vi "PTFE Test.vi"() -> ()   [LabVIEW 2015]
uses:
  Controls/Vacuum State Enumerator.ctl
  <vilib>/Platform/TimedLoop/XDataNode/timing_clust.ctl
  <vilib>/Platform/TimedLoop/XDataNode/nitl_modes.ctl
  <vilib>/Platform/TimedLoop/XDataNode/wakeup.ctl
  <vilib>/platform/TimedLoop/XDataNode/XDataNode.xnode
  <vilib>/Platform/TimedLoop/XDataNode/XDNodeRunTimeDep.lvlib
panel:
  out "x/y":dbl(slide) scale=0.0..1.0
  in  "Enable":bool
  in  "Waveform Graph 3":dbl[](graph)=array[50278 elements]
  out "Waveform Graph 2":dbl[](graph)
  in  "Vacuum State":T1=enum."Unknown"
  out "Valve":bool
  in  "Numeric":dbl
  out "Waveform Graph":dbl[](graph)
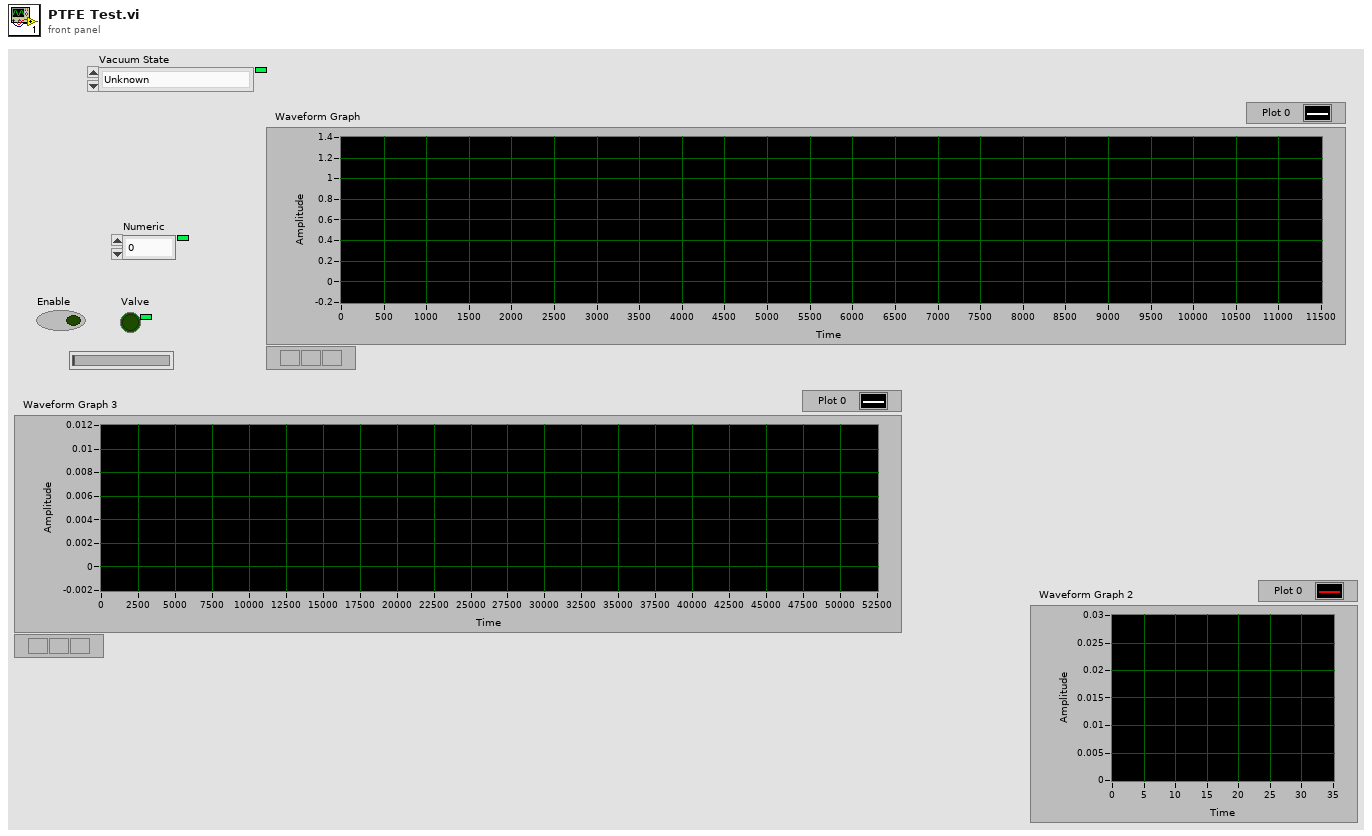
[diagram p1: front panel]
types:
  T1 = typedef "Vacuum State Enumerator.ctl" = enum16{"Pressure Rising", "Plateau", "Pressure Dropping", "Valley", "Low Valley", "Leak", "Unknown"}
  T2 = typedef "XDNodeRunTimeDep.lvlib/timing_clust.ctl" = cluster{"Expected End [f-1]":u64, "Actual End [f-1]":u64, "Finished Late? [f-1]":bool, "Expected End [i-1]":u64, "Actual End [i-1]":u64, "Finished Late? [i-1]":bool, "Expected Start [i]":u64, "Actual Start [i]":u64, "Expected Start [f]":u64, "Actual Start [f]":u64, "Source Name":string, "Structure Name":string, "Period":i64, "Deadline":i64, "Offset":i64, "Start":i64, "Priority":i32, "Timeout":i32, "Mode":T3, "Wakeup Reason":T4, "Error":errorcluster, "Source Type":string, "Secondary Source Type":string, "Global End Time":u64, "Global Start Time":u64, "Frame Duration":u64, "Iteration Duration":u64, "Assigned CPU":i32, "I/O Scan Engine Mode":u32}
  T3 = typedef "XDNodeRunTimeDep.lvlib/nitl_modes.ctl" = enum32{"No Change", "Process missed periods, maintain original phase", "Discard missed periods, maintain original phase", "Process missed periods, ignore original phase", "Discard missed periods, ignore original phase"}
  T4 = typedef "XDNodeRunTimeDep.lvlib/wakeup.ctl" = enum32{"Normal", "Aborted", "Asynchronous wakeup", "Timing source error", "Timed loop error", "Timeout"}
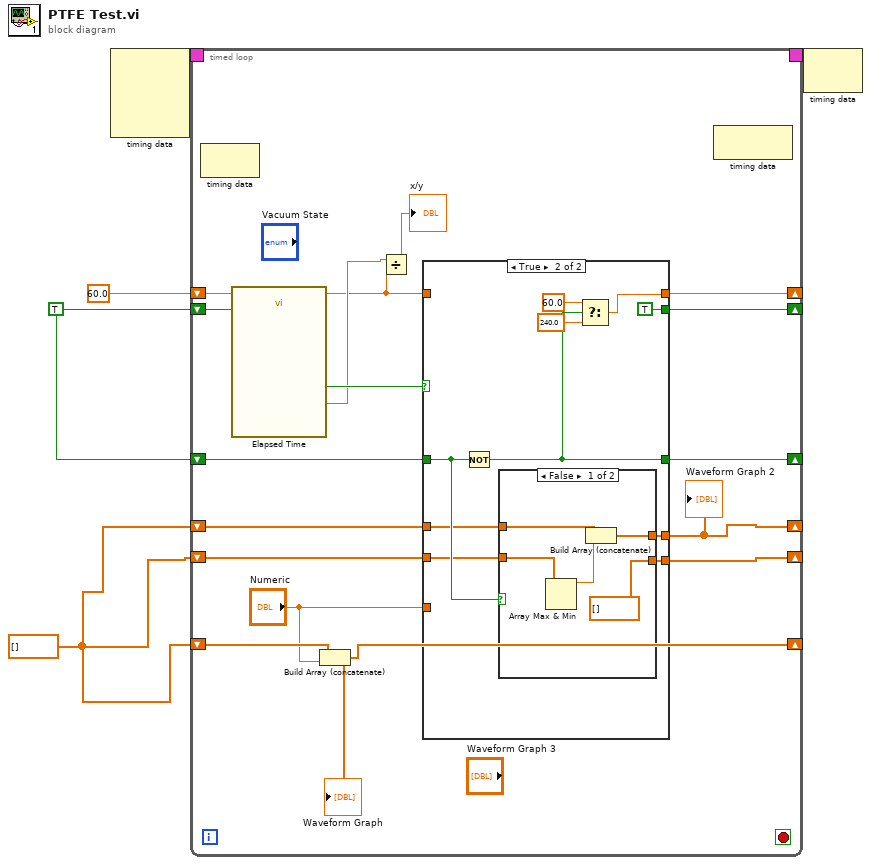
[diagram p0: block diagram]
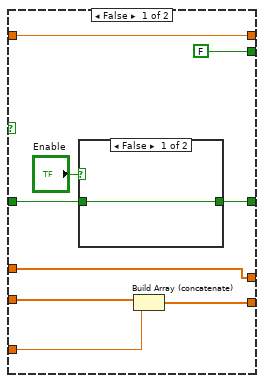
[diagram p2: hidden frame]
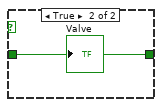
[diagram p3: hidden frame]
diagram:
  w1 = dbl[] []
  w2 = TRUE
  n1 = node-c288() -> (w5:T2)  [unwired: 4 in]
  n2 = timed-loop {
    timing: w5 -> [_]
    timing-out: [_] -> w4
    shift-right: [w15] -> _
    shift-left: w2 -> [w21]
    shift-right: [w19] -> _
    shift-left: w1 -> [w20]
    shift-right: [w14] -> _
    shift-left: 60.0 -> [w7]
    shift-right: [w16] -> _
    shift-left: w2 -> [w18]
    shift-right: [w11] -> _
    shift-left: w1 -> [w13]
    shift-right: [w10] -> _
    shift-left: w1 -> [w12]
    stop <- _ stop-if-true
    n3 = node-c288() -> ()  [unwired: 1 in, 1 out]
    n4 = call "Elapsed Time"("Time Target (s)"=w7, "Reset"=w21) -> ("Elapsed Time (s)"=w8:dbl, "Time has Elapsed"=w17:bool)  [unwired: 10 in, 6 out]
    n5 = Build Array (concatenate)(w20, "Numeric") -> (w19:dbl[])
    "Waveform Graph" <- w19
    n6 = Divide(x=w8, y=w7) -> (x/y=→"x/y":dbl)
    n7 = case shown="True" w17 {
      tunnel: w18 -> [w30 w37]
      tunnel: [w22 w41] -> w16
      tunnel: [FALSE TRUE] -> w15
      tunnel: [w28 w38] -> w14
      tunnel: w7 -> [w28 _]
      tunnel: "Numeric" -> [w26 _]
      tunnel: w13 -> [w27 w36]
      tunnel: w12 -> [w24 w35]
      tunnel: [w24 w34] -> w10
      tunnel: [w25 w33] -> w11
      frame False {
        n8 = case shown="False" "Enable" {
          tunnel: w30 -> [w31 w32]
          tunnel: [w31 w32] -> w22
          frame False {
          }
          frame True {
            "Valve" <- w32
          }
        }
        n9 = Build Array (concatenate)(w27, w26) -> (w25:dbl[])
      }
      frame True {
        n10 = Not(x=w37) -> (.not. x?=w41:bool)
        n11 = case shown="False" w37 {
          tunnel: w36 -> [w47 _]
          tunnel: w35 -> [w46 w48]
          tunnel: [w44 w48] -> w34
          tunnel: [dbl[] [] _] -> w33
          frame False {
            n12 = Array Max & Min(array=w47) -> (max value=w45:dbl)  [unwired: 3 out]
            n13 = Build Array (concatenate)(w46, w45) -> (w44:dbl[])
          }
          frame True {
          }
        }
        n14 = Select(t=60.0, s=w41, f=240.0) -> (s? t:f=w38:dbl)
      }
    }
    "Waveform Graph 2" <- w10
    n15 = node-c288() -> ()  [unwired: 1 in, 1 out]
  }
  n16 = node-c288(w4) -> ()  [unwired: 1 out]
